vi "DiagnosticCheckMain.vi"(0 "CameraControllerParameters.Diagnostics":T1, 5 "Diagnostic Check Image":T2, 11 "error in (no error)":errorcluster) -> (4 "Diagnostics Passed":bool, 6 "Diagnostic Check Image out":T2, 10 "Dust Percentage":dbl, 14 "Diagnostics status":string, 15 "error out":errorcluster)   [LabVIEW 2019]
uses:
  <vilib>/vision/Image Controls.llb/IMAQ Image.ctl
  Camera Controller/Camera Controller Actor/TypeDef/CameraControllerParameters.ctl
  Camera Controller/Camera Controller Actor/Camera Controller.lvclass
panel:
  out "Image Pixels (U8) 2":u8[][](array[numeric])
  in  "Image Pixels (U8)":u8[][](array[numeric])
  in  "File Path":path
  in  "Offline":bool
  out "Waveform Graph":u32[](graph)
  out "Range Percentage":dbl[](array[numeric])
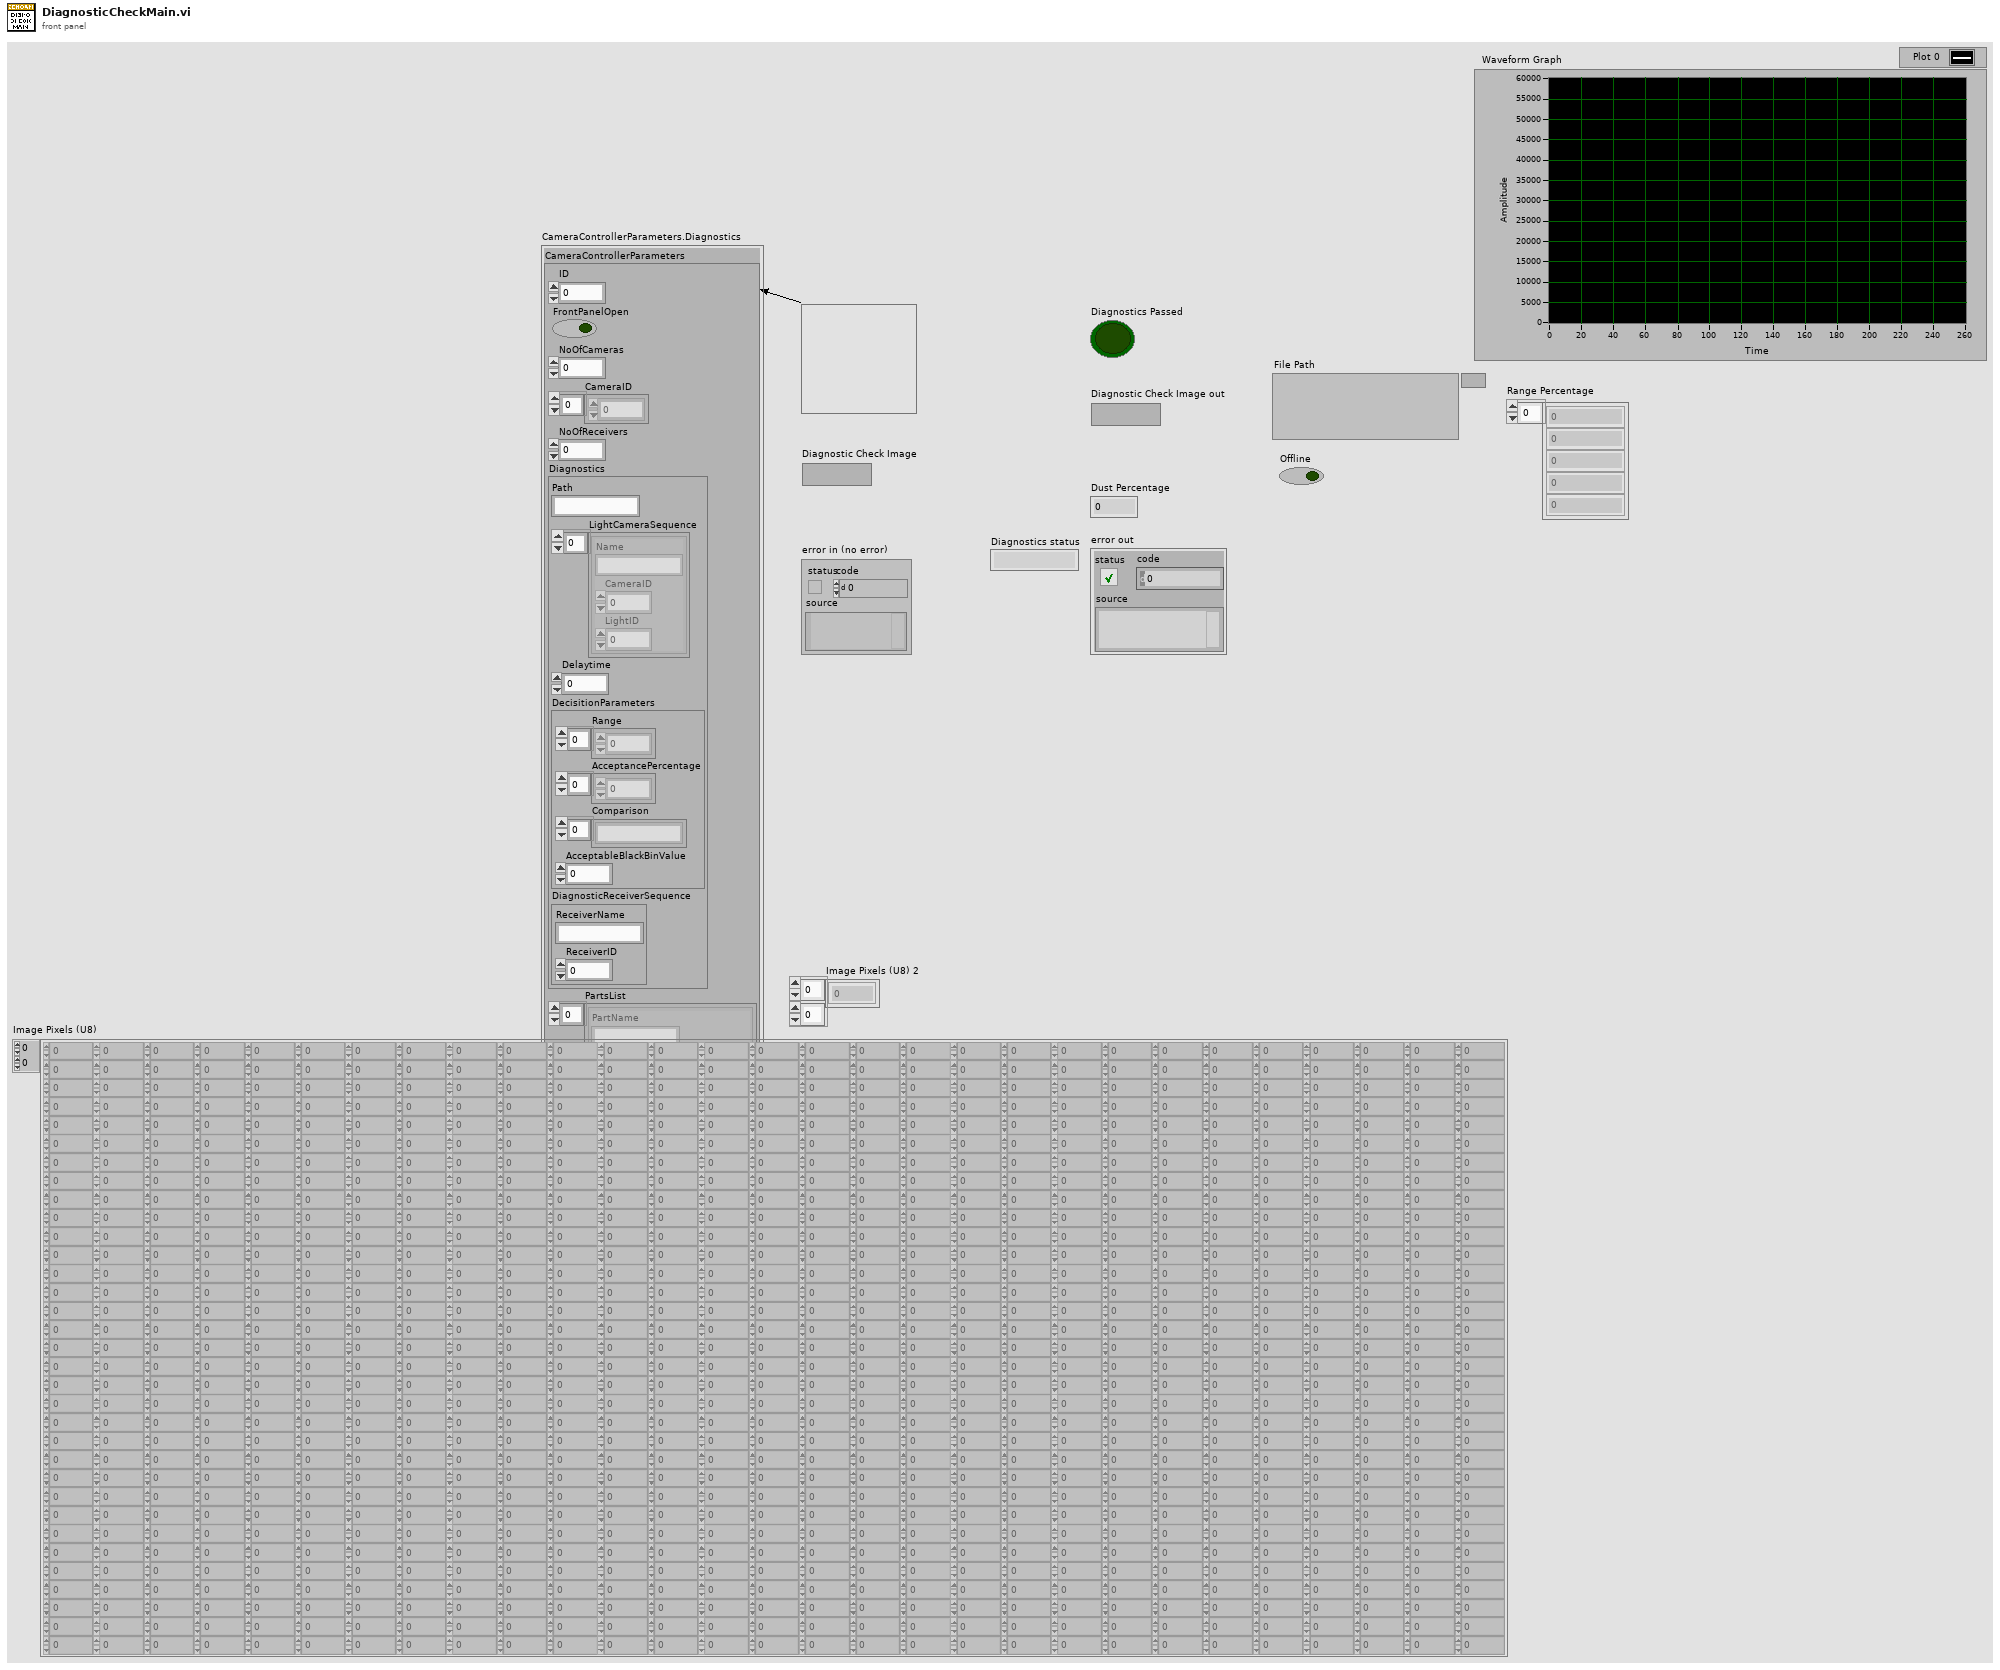
[diagram p1: front panel]
types:
  T1 = typedef "Camera Controller.lvlib/Camera Controller.lvclass/CameraControllerParameters.ctl" = cluster{"CameraControllerParameters":cluster{"ID":i32, "FrontPanelOpen":bool, "NoOfCameras":i32, "CameraID":i32[], "NoOfReceivers":i32, "Diagnostics":cluster{"Path":string, "LightCameraSequence":cluster{"Name":string, "CameraID":i32, "LightID":i32}[], "Delaytime":dbl, "DecisitionParameters":cluster{"Range":i32[], "AcceptancePercentage":i32[], "Comparison":string[], "AcceptableBlackBinValue":i32}, "DiagnosticReceiverSequence":cluster{"ReceiverName":string, "ReceiverID":i32}}, "PartsList":cluster{"PartName":string, "CameraIDs":i32[], "ReceiverSequence":cluster{"ReceiverName":string, "ReceiverID":i32, "NoOfActiveCameras":i32}[]}[]}, "PartName":string[]}
  T2 = typedef "IMAQ Image.ctl" = refnum<image>
  T3 = cluster{"histogram":u32[], "Minimal Value":sgl, "Maximal Value":sgl, "Starting Value":sgl, "Interval Width":sgl, "Mean Value":sgl, "Standard  Variation":sgl, "Area (pixels)":i32}
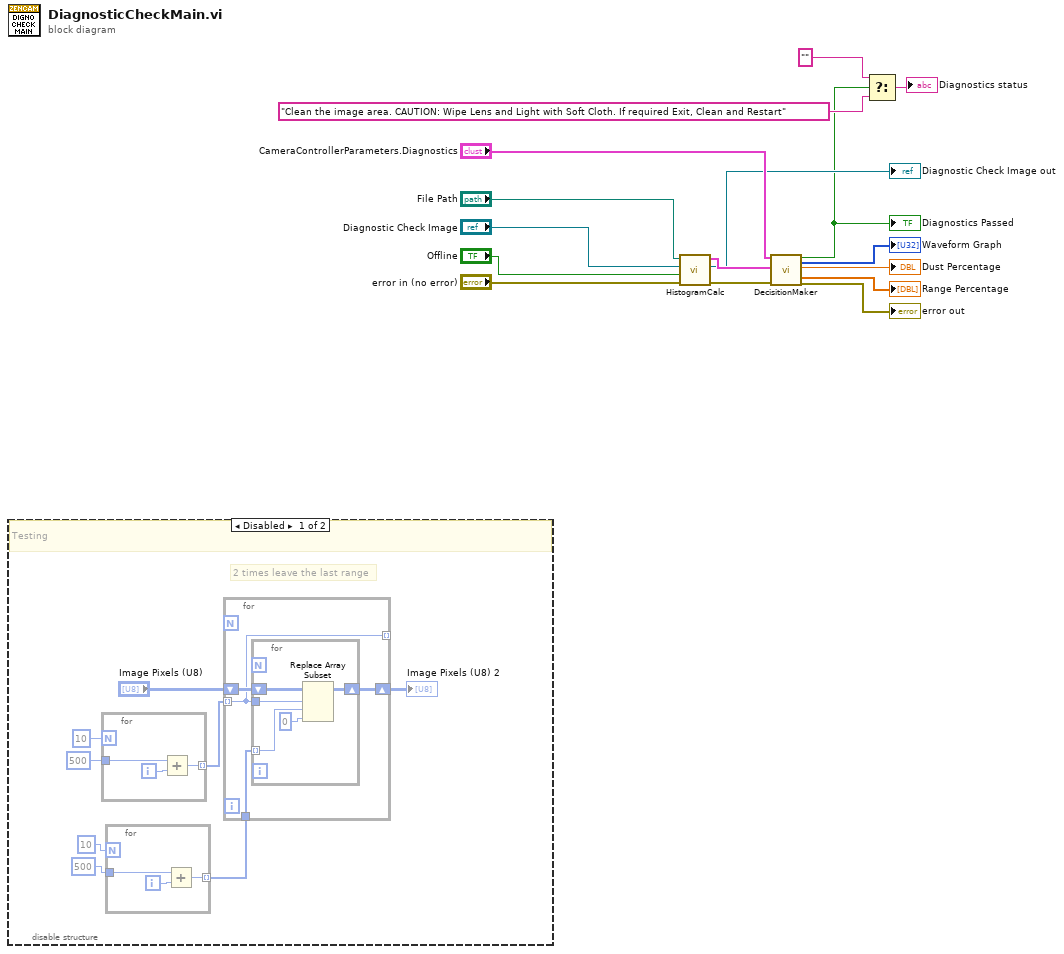
[diagram p0: block diagram]
diagram:
  n1 = disable-structure shown="Disabled" {
    frame Disabled {
      # "2 times leave the last range"
      # "Testing"
      n2 = for {
        N: 10 -> [_]
        tunnel: 500 -> [w30]
        tunnel: [w28] -> w20 mode=indexing
        i -> [w29]
        n3 = Add(x=w30, y=w29) -> (x+y=w28:i32)
      }
      n4 = for {
        N: 10 -> [_]
        tunnel: 500 -> [w27]
        tunnel: [w25] -> w17 mode=indexing
        i -> [w26]
        n5 = Add(x=w27, y=w26) -> (x+y=w25:i32)
      }
      n6 = for {
        shift-right: [w33] -> w23
        shift-left: "Image Pixels (U8)" -> [w34]
        tunnel: [w32] -> _ mode=indexing
        tunnel: w20 -> [w32] mode=indexing
        tunnel: w17 -> [w31]
        n7 = for {
          tunnel: w32 -> [w36]
          tunnel: w31 -> [w35] mode=indexing
          shift-right: [w38] -> w33
          shift-left: w34 -> [w39]
          n8 = Replace Array Subset(array=w39, new element=u8 0 ("new element/subarray"), index (row)=w36, index (col)=w35) -> (w38:u8[][])
        }
      }
      "Image Pixels (U8) 2" <- w23
    }
    frame Enabled {
    }
  }
  n9 = call "HistogramCalc.vi"("error in (no error)"="error in (no error)", "Offline"="Offline", "Diagnostic Check Image"="Diagnostic Check Image", "File Path"="File Path") -> ("error out"=w15:errorcluster, "Image Out"=→"Diagnostic Check Image out":T2, "Histogram Report"=w16:T3)  [unwired: 5 in]
  n10 = call "DecisitionMaker.vi"("CameraControllerParameters.Diagnostics"="CameraControllerParameters.Diagnostics", "Histogram Report"=w16, "error in (no error)"=w15) -> ("Diagnostics Passed"=w1:bool, "Waveform Graph"=→"Waveform Graph":u32[], "Dust Percentage"=→"Dust Percentage":dbl, "Range Percentage"=→"Range Percentage":dbl[], "error out"=→"error out":errorcluster)  [unwired: 10 in, 2 out]
  "Diagnostics Passed" <- w1
  n11 = Select(t="" ("status"), s=w1, f="Clean the image area. CAUTION: Wipe Lens and Light with Soft Cloth. If required Exit, Clean and Restart" ("status")) -> (s? t:f=→"Diagnostics status":string)
